vi "猜数程序while.vi"() -> ()   [LabVIEW 2014]
panel:
  out "字符串":string
  in  "数值":dbl
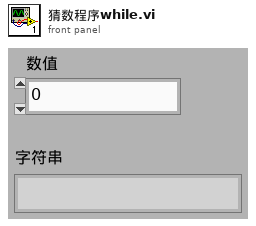
[diagram p1: front panel]
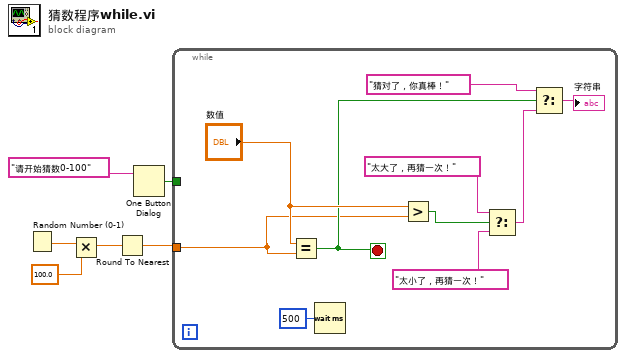
[diagram p0: block diagram]
diagram:
  n1 = Random Number (0-1)() -> (number: 0 to 1=w4:dbl)
  n2 = Multiply(x=w4, y=100.0) -> (x*y=w2:dbl)
  n3 = Round To Nearest(number=w2) -> (nearest integer value=w1:dbl)
  n4 = One Button Dialog(message="请开始猜数0-100" ("消息")) -> (true=w6:bool)  [unwired: 1 in]
  n5 = while {
    tunnel: w6 -> [_]
    tunnel: w1 -> [w7]
    stop <- w11 stop-if-true
    n6 = Equal?(x="数值", y=w7) -> (x = y?=w11:bool)
    n7 = Wait (ms)(milliseconds to wait=u32 500 ("等待时间（毫秒）")) -> ()  [unwired: 1 out]
    n8 = Greater?(x="数值", y=w7) -> (0:w12:bool)
    n9 = Select(t="太大了，再猜一次！", s=w12, f="太小了，再猜一次！") -> (s? t:f=w8:string)
    n10 = Select(t="猜对了，你真棒！" ("f"), s=w11, f=w8) -> (s? t:f=→"字符串":string)
  }
